vi "Validate Channel Name.vi"(8 "error in (no error)":errorcluster, 10 "Name In":string, 11 "Refnum In":T1 format="%.0x") -> (0 "error out":errorcluster, 2 "Name Out":string, 3 "Refnum Out":T1 format="%.0x")   [LabVIEW 2020, in "Instrument Addon Scripting API.lvlib"]
uses:
  Instrument Addon Scripting API.lvlib
  <vilib>/NI VeriStand/Custom Device API/Custom Device Item Ref.ctl
  <vilib>/NI VeriStand/Custom Device Tools/Custom Device Utility Library/Custom Device Utility Library.lvlib
  <vilib>/NI VeriStand/Custom Device API/Custom Device API.lvlib
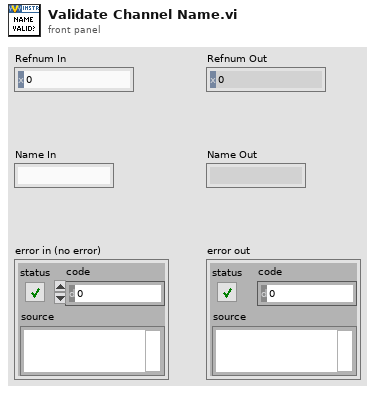
[diagram p1: front panel]
types:
  T1 = typedef "Custom Device API.lvlib/Custom Device Item Ref.ctl" = u64
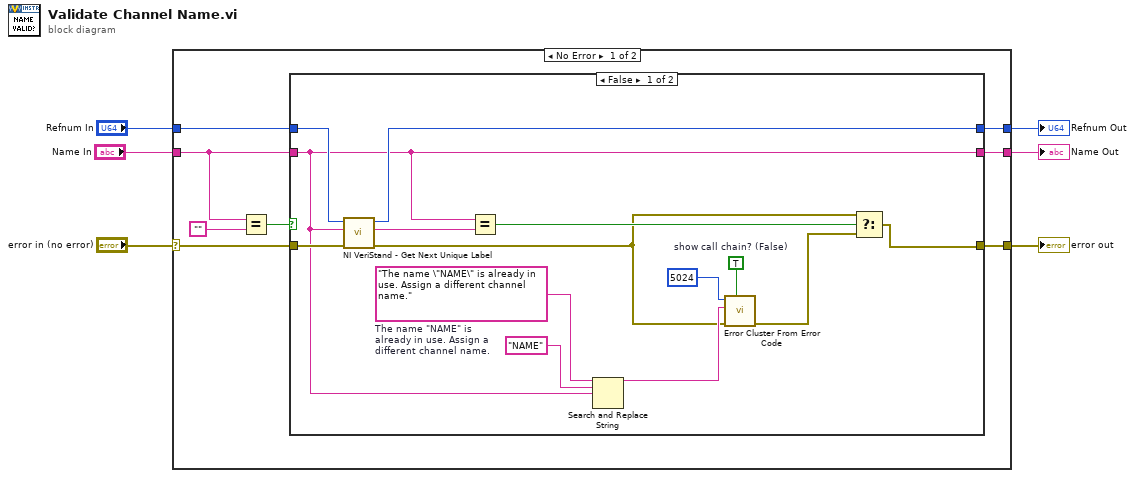
[diagram p0: block diagram]
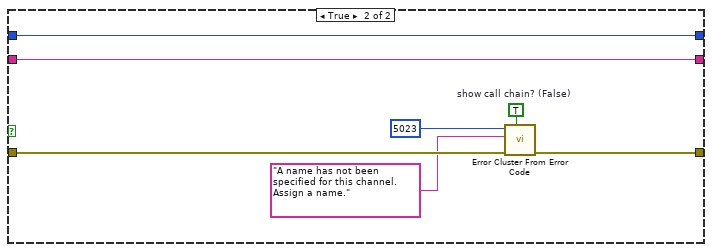
[diagram p2: hidden frame]
diagram:
  n1 = case shown="No Error" "error in (no error)" {
    selector: "error in (no error)" -> [w7 w38]
    tunnel: [w14 w37] -> w6
    tunnel: [w13 w38] -> w5
    tunnel: "Refnum In" -> [w12 w37]
    tunnel: "Name In" -> [w9 w36]
    tunnel: [w8 w36] -> w2
    frame No Error {
      n2 = Equal?(x=w9, y="") -> (x = y?=w10:bool)
      n3 = case shown="False" w10 {
        tunnel: [w28 w35] -> w14
        tunnel: [w17 w33] -> w13
        tunnel: w7 -> [w27 w31]
        tunnel: w12 -> [w26 w35]
        tunnel: w9 -> [w22 w34]
        tunnel: [w22 w34] -> w8
        frame False {
          w19 = TRUE  # show call chain? (False)
          w23 = "The name \"NAME\" is already in use. Assign a different channel name."  # The name "NAME" is already in use. Assign a different channel name.
          n4 = call <vilib>:"NI VeriStand - Get Next Unique Label.vi"("error in (no error)"=w27, "Label"=w22, "Parent Ref in"=w26) -> ("error out"=w15:errorcluster, "Label out"=w25:string, "Parent Ref dup"=w28:T1)  [unwired: 5 in, 1 out]
          n5 = Equal?(x=w22, y=w25) -> (x = y?=w18:bool)
          n6 = Search and Replace String(input string=w23, search string="NAME", replace string=w22) -> (result string=w20:string)  [unwired: 5 in, 3 out]
          n7 = call <vilib>:"Error Cluster From Error Code.vi"("show call chain? (False)"=w19, "error in (no error)"=w15, "error message (\"\")"=w20, "error code (0)"=5024 ("code")) -> ("error out"=w16:errorcluster)  [unwired: 5 in]
          n8 = Select(t=w15, s=w18, f=w16) -> (s? t:f=w17:errorcluster)
        }
        frame True {
          w29 = TRUE  # show call chain? (False)
          n9 = call <vilib>:"Error Cluster From Error Code.vi"("show call chain? (False)"=w29, "error in (no error)"=w31, "error message (\"\")"="A name has not been specified for this channel. Assign a name." ("error message (\"\")"), "error code (0)"=5023) -> ("error out"=w33:errorcluster)  [unwired: 5 in]
        }
      }
    }
    frame Error {
    }
  }
  "Refnum Out" <- w6
  "error out" <- w5
  "Name Out" <- w2
